vi "Wait.vi"(8 "error in (no error)":errorcluster, 10 "Timeout in ms (0)":i32, 11 "Sequencer Core in":refnum<class "Sequencer Core.lvclass">) -> (0 "error out":errorcluster, 1 "Timed out?":bool, 3 "Sequencer Core out":refnum<class "Sequencer Core.lvclass">)   [LabVIEW 2020, in "Sequencer.lvlib" / "Sequencer Core.lvclass"]
doc: "Wait for interrupt on the Interrupt Notifier."
uses:
  Sequencer Core.lvclass
  Sequencer Core.lvclass/Sequencer Core.ctl
  PPL/HDH.Data.Generic.lvlibp/Synchronization/Notifier/Notifier.lvclass
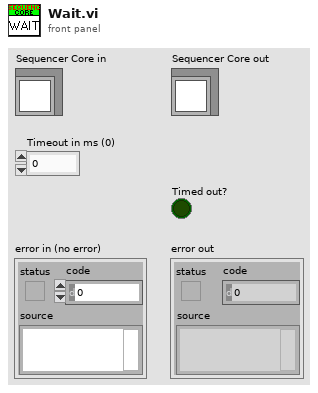
[diagram p1: front panel]
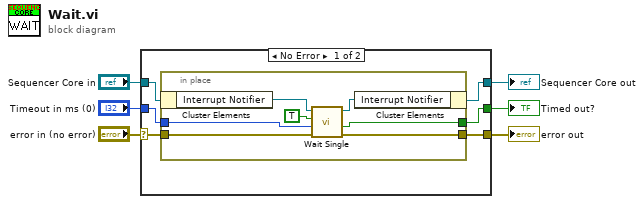
[diagram p0: block diagram]
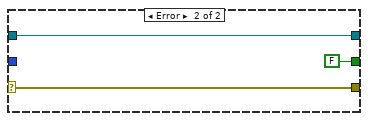
[diagram p2: hidden frame]
diagram:
  n1 = case shown="No Error" "error in (no error)" {
    selector: "error in (no error)" -> [w9 w22]
    tunnel: [w8 w22] -> w5
    tunnel: [w10 w21] -> w3
    tunnel: "Sequencer Core in" -> [w12 w21]
    tunnel: "Timeout in ms (0)" -> [w11 _]
    tunnel: [w7 FALSE ("Timed out?")] -> w1
    frame No Error {
      n2 = in-place {
        in-place-border: w11 -> [w19]
        in-place-border: w9 -> [w18]
        in-place-border: [w14] -> w8
        in-place-border: [w13] -> w7
        n3 = in-place-cluster #1(w12) -> ("Interrupt Notifier"=w17:refnum<class "Notifier.lvclass">)
        n4 = call "Wait Single.vi"("error in (no error)"=w18, "Timeout in ms (-1)"=w19, "Ignore previous (F)"=TRUE, "Notifier in"=w17) -> ("error out"=w14:errorcluster, "Timed out?"=w13:bool, "Notifier out"=w16:refnum<class "Notifier.lvclass">)  [unwired: 4 in, 1 out]
        n5 = in-place-cluster #1("Interrupt Notifier"=w16) -> (w10:refnum<class "Sequencer Core.lvclass">)
      }
    }
    frame Error {
    }
  }
  "error out" <- w5
  "Sequencer Core out" <- w3
  "Timed out?" <- w1
